vi "Set_speed_and_move_XY_set_local_origin.vi"() -> ()   [LabVIEW 2013]
panel:
  out "Received String2 3":string="R\r\n"
  out "Received String1":string="OK\r\n"
  out "OK Done":bool=TRUE
  out "Received String2 2":string="R\r\n"
  out "String Received 4":string="OK\r\n"
  out "Command String 4":string="A:2+P10000"
  out "OK move 2":bool=TRUE
  in  "Pulse Number 2":u32=80000 min=1 max=500000
  in  "Axis Number 2":u8=2
  out "OK speed 2":bool=TRUE
  out "String Received 3":string="OK\r\n"
  out "Command String 3":string="D:2S1000F40000R100"
  in  "Acceleration Time 2":u16=100 max=1000
  in  "High Speed 2":u32=40000 min=1 max=500000
  in  "Low Speed 2":u32=1000 min=1 max=500000
  out "Received String2":string="R\r\n"
  out "String Received 2":string="OK\r\n"
  out "Command String 2":string="A:1+P10000"
  out "OK move 1":bool=TRUE
  in  "Pulse Number 1":u32=1 min=1 max=500000
  in  "Axis Number 1":u8=1
  out "OK speed 1":bool=TRUE
  in  "Port Number":i8=10 min=0
  out "String Received":string="OK\r\n"
  out "Command String":string="D:1S1000F40000R100"
  in  "Acceleration Time":u16=100 max=1000
  in  "High Speed":u32=40000 min=1 max=500000
  in  "Low Speed":u32=1000 min=1 max=500000
  # "For tensile test (30 mm sample length):\nSet local origin as X (axis 1) 27000, Y (axis 2) 5000"
  # "Set speed"
  # "Move to the absolute position"
  # "Abs. position X\nin um"
  # "X"
  # "Abs. position Y\nin um"
  # "Y"
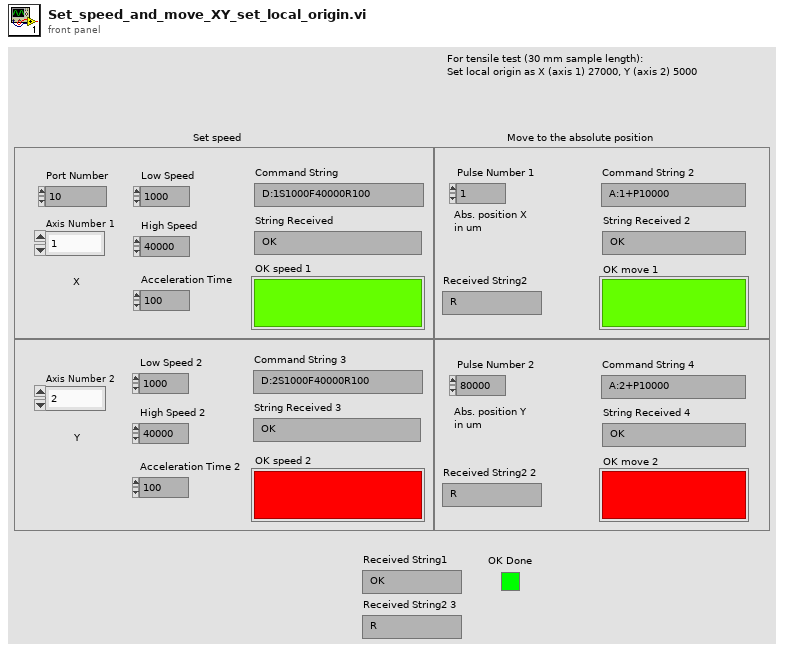
[diagram p1: front panel]
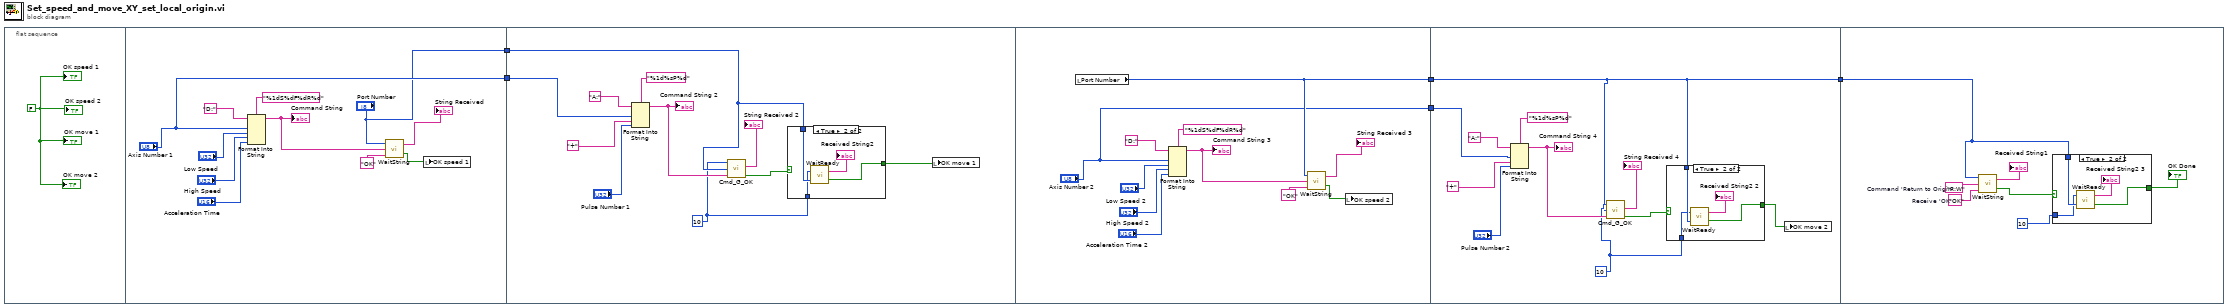
[diagram p0: block diagram]
diagram:
  n1 = flat-sequence {
    tunnel: ["Axis Number 1"] -> w5
    tunnel: ["Port Number"] -> w4
    tunnel: w5 -> [w21]
    tunnel: w4 -> [w20]
    tunnel: [w36] -> w3
    tunnel: ["Axis Number 2"] -> w2
    tunnel: w3 -> [w45]
    tunnel: w2 -> [w48]
    tunnel: [w45] -> w1
    tunnel: w1 -> [w61]
    frame #0 {
      w6 = FALSE
      "OK speed 1" <- w6
      "OK speed 2" <- w6
      "OK move 1" <- w6
      "OK move 2" <- w6
    }
    frame #1 {
      n2 = Format Into String(format string="%1dS%dF%dR%d", initial string="D:", "Axis Number 1", "Low Speed", "High Speed", "Acceleration Time") -> (resulting string=w11:string)  [unwired: 1 in, 1 out]
      "Command String" <- w11
      n3 = call "WaitString.vi"("String to Receive"="OK", "String to Send"=w11, "PortNumber"="Port Number") -> ("OK Done"=w7:bool, "String Received"=→"String Received":string)
      n4 = local write "OK speed 1"(w7) -> ()
    }
    frame #2 {
      w18 = 10
      n5 = Format Into String(format string="%1d%sP%d", initial string="A:", w21, "+", "Pulse Number 1") -> (resulting string=w25:string)  [unwired: 1 in, 1 out]
      "Command String 2" <- w25
      n6 = call "Cmd_G_OK.vi"("Residence time"=w18, "PortNumber"=w20, "Command String"=w25) -> ("Received String2"=→"String Received 2":string, "OK Done"=w27:bool)  [unwired: 2 out]
      n7 = case shown="True" w27 {
        selector: w27 -> [w29 _]
        tunnel: w20 -> [_ w33]
        tunnel: [w29 w31] -> w19
        tunnel: w18 -> [_ w30]
        frame False {
        }
        frame True {
          n8 = call "WaitReady.vi"("PortNumber"=w33, "Residence time in ms"=w30) -> ("OK Done"=w31:bool, "String Received"=→"Received String2":string)
        }
      }
      n9 = local write "OK move 1"(w19) -> ()
    }
    frame #3 {
      n10 = local read "Port Number"() -> (w36:i8)
      n11 = Format Into String(format string="%1dS%dF%dR%d", initial string="D:", "Axis Number 2", "Low Speed 2", "High Speed 2", "Acceleration Time 2") -> (resulting string=w43:string)  [unwired: 1 in, 1 out]
      "Command String 3" <- w43
      n12 = call "WaitString.vi"("String to Receive"="OK", "String to Send"=w43, "PortNumber"=w36) -> ("OK Done"=w34:bool, "String Received"=→"String Received 3":string)
      n13 = local write "OK speed 2"(w34) -> ()
    }
    frame #4 {
      w46 = 10
      n14 = Format Into String(format string="%1d%sP%d", initial string="A:", w48, "+", "Pulse Number 2") -> (resulting string=w52:string)  [unwired: 1 in, 1 out]
      "Command String 4" <- w52
      n15 = call "Cmd_G_OK.vi"("Residence time"=w46, "PortNumber"=w45, "Command String"=w52) -> ("Received String2"=→"String Received 4":string, "OK Done"=w50:bool)  [unwired: 2 out]
      n16 = case shown="True" w50 {
        selector: w50 -> [w56 _]
        tunnel: [w56 w59] -> w47
        tunnel: w45 -> [_ w58]
        tunnel: w46 -> [_ w57]
        frame False {
        }
        frame True {
          n17 = call "WaitReady.vi"("PortNumber"=w58, "Residence time in ms"=w57) -> ("OK Done"=w59:bool, "String Received"=→"Received String2 2":string)
        }
      }
      n18 = local write "OK move 2"(w47) -> ()
    }
    frame #5 {
      w67 = "OK"  # Receive 'OK'
      w66 = "R:W"  # Command 'Return to Origin'
      n19 = call "WaitString.vi"("String to Receive"=w67, "String to Send"=w66, "PortNumber"=w61) -> ("OK Done"=w64:bool, "String Received"=→"Received String1":string)
      n20 = case shown="True" w64 {
        selector: w64 -> [w68 _]
        tunnel: w61 -> [_ w72]
        tunnel: [w68 w70] -> w62
        tunnel: 10 -> [_ w69]
        frame False {
        }
        frame True {
          n21 = call "WaitReady.vi"("PortNumber"=w72, "Residence time in ms"=w69) -> ("OK Done"=w70:bool, "String Received"=→"Received String2 3":string)
        }
      }
      "OK Done" <- w62
    }
  }
